vi "PFI-28000-Card_Get Test Mode Options.vi"(8 "error in (no error)":errorcluster, 11 "PFI-28000-Card in":refnum<class "PFI-28000-Card.lvclass">) -> (0 "error out":errorcluster, 2 "Options":string[](array[string]), 3 "PFI-28000-Card out":refnum<class "PFI-28000-Card.lvclass">)   [LabVIEW 2017, in "PFI-28000-Card.lvclass"]
uses:
  PFI-28000-Card.lvclass
  PFI-28000-Card.lvclass/PFI-28000-Card.ctl
  Channel/PFI-28000-Channel.lvclass
  Utilities/PFI-28000-Utils.lvlib
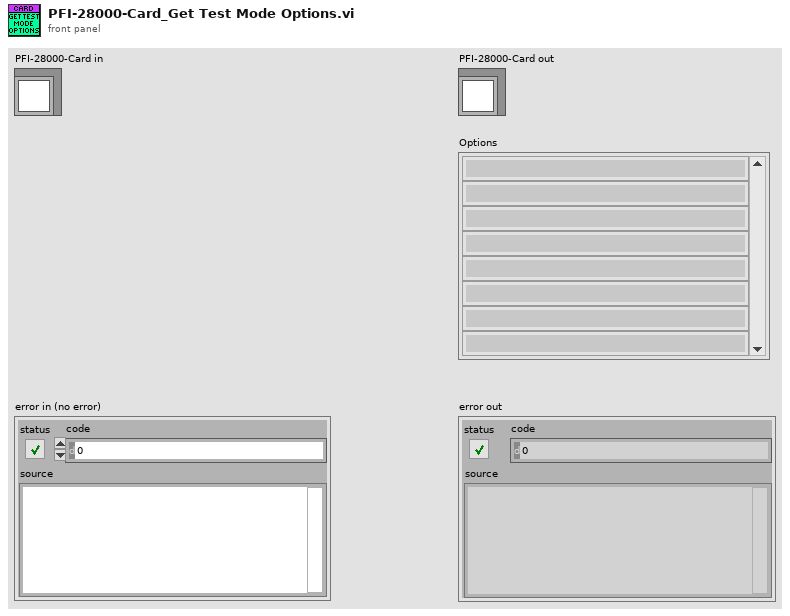
[diagram p1: front panel]
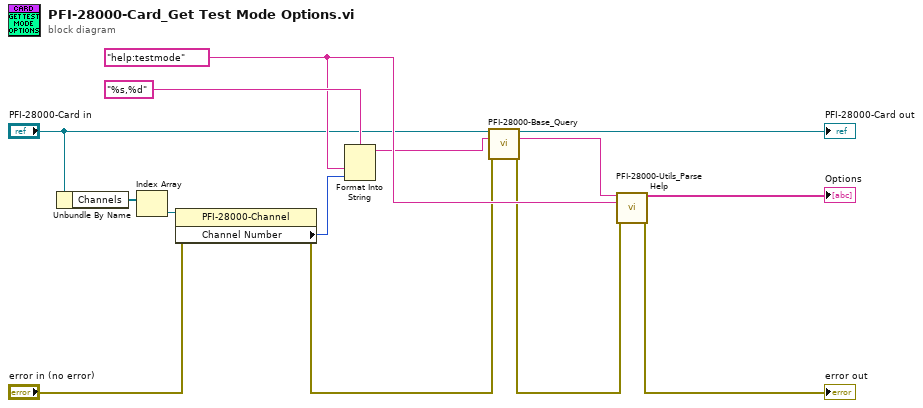
[diagram p0: block diagram]
diagram:
  w7 = "help:testmode" ("empty string")
  n1 = Unbundle By Name("PFI-28000-Card in") -> ("Channels"=w11:refnum<class "PFI-28000-Channel.lvclass">[])
  n2 = Index Array(array=w11) -> (element=w10:refnum<class "PFI-28000-Channel.lvclass">)  [unwired: 1 in]
  n3 = property class="PFI-28000-Channel"(reference=w10, error in="error in (no error)") -> (error out=w3:errorcluster, "Channel Number"=w13:i32)  [unwired: 1 out]
  n4 = Format Into String(format string="%s,%d" ("empty string"), w7, w13) -> (resulting string=w4:string)  [unwired: 2 in, 1 out]
  n5 = call-dynamic "PFI-28000-Base_Query.vi"("PFI-28000-Base in"="PFI-28000-Card in", "Command"=w4, "error in (no error)"=w3) -> ("PFI-28000-Base out"=→"PFI-28000-Card out":refnum<class "PFI-28000-Card.lvclass">, "Response"=w1:string, "error out"=w2:errorcluster)  [unwired: 9 in, 1 out]
  n6 = call "PFI-28000-Utils_Parse Help.vi"("String"=w1, "Command"=w7, "error in (no error)"=w2) -> ("Options"=→"Options":string[], "error out"=→"error out":errorcluster)  [unwired: 11 in]
